vi "Wait for Operation Complete.vi"(2 "error in (no error)":errorcluster, 3 "Timeout (10000 ms)":u32=10000, 4 "VISA resource name":refnum<visa-resource-name>) -> (0 "error out":errorcluster, 1 "VISA resource name out":refnum<visa-resource-name>)   [LabVIEW 2020]
doc: "This low-level VI initiates a measurement. After you call this VI, the instrument leaves the idle state and waits for a trigger.\n\n<B>Note:</B> Use this VI only with other low-level VIs. The high-level VIs automatically incorporate this functionality. This VI does not check the instrument status. If you want to check the instrument status, call the Error Query VI at the conclusion of the sequence."
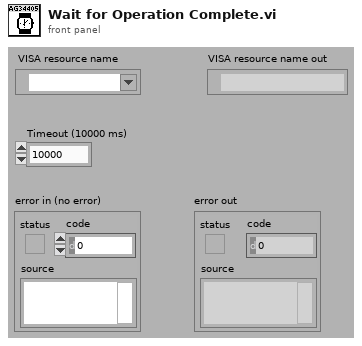
[diagram p1: front panel]
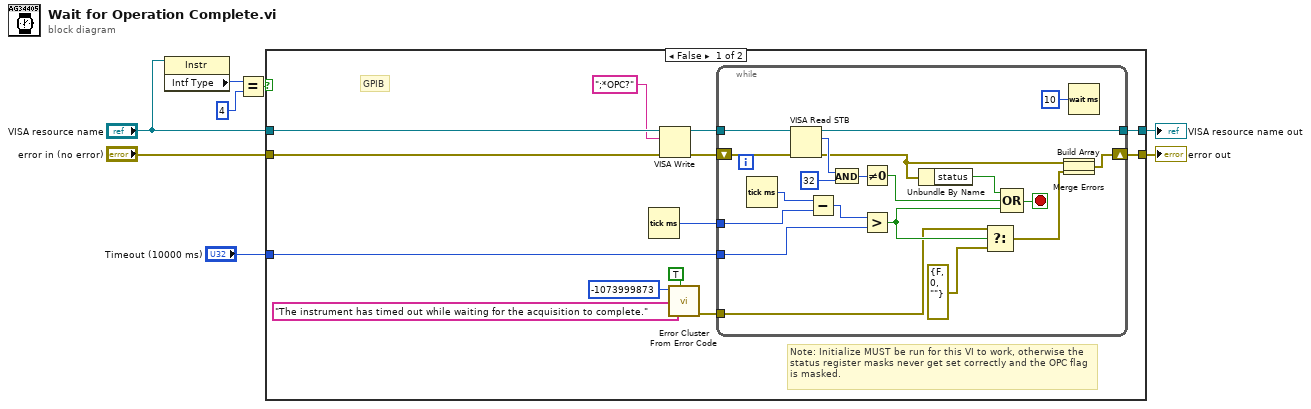
[diagram p0: block diagram]
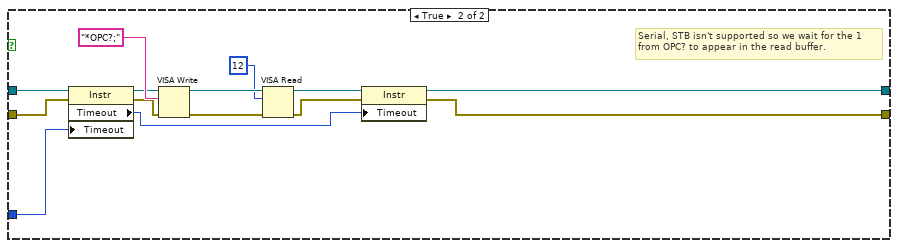
[diagram p2: hidden frame]
diagram:
  n1 = property class="Instr"(reference="VISA resource name") -> ("Intf Type"=w3:u16)  [unwired: 1 in, 2 out]
  n2 = Equal?(x=w3, y=u16 4) -> (x = y?=w4:bool)
  n3 = case shown="False" w4 {
    tunnel: "VISA resource name" -> [w21 w52]
    tunnel: "error in (no error)" -> [w20 w47]
    tunnel: [w17 w43] -> w7
    tunnel: [w16 w48] -> w6
    tunnel: "Timeout (10000 ms)" -> [w9 w51]
    frame False {
      # "GPIB"
      # "Note: Initialize MUST be run for this VI to work, otherwise the status register masks never get set correctly and the OPC flag is masked."
      n4 = Tick Count (ms)() -> (millisecond timer value=w14:u32)
      n5 = VISA Write(VISA resource name=w21, write buffer=";*OPC?", error in (no error)=w20) -> (VISA resource name out=w19:refnum<visa-resource-name>, error out=w18:errorcluster)  [unwired: 1 out]
      n6 = call <vilib>:"Error Cluster From Error Code.vi"("show call chain? (False)"=TRUE, "error message (\"\")"="The instrument has timed out while waiting for the acquisition to complete." ("error message (\"\")"), "error code (0)"=-1073999873) -> ("error out"=w10:errorcluster)  [unwired: 6 in]
      n7 = while {
        tunnel: w19 -> [w42]
        tunnel: [w40] -> w16
        tunnel: w14 -> [w35]
        shift-right: [w27] -> w17
        shift-left: w18 -> [w41]
        tunnel: w10 -> [w30]
        tunnel: w9 -> [w23]
        stop <- w32 stop-if-true
        n8 = Tick Count (ms)() -> (millisecond timer value=w36:u32)
        n9 = VISA Read STB(8:w41, 11:w42) -> (0:w26:errorcluster, 2:w39:u16, 3:w40:refnum<visa-resource-name>)
        n10 = Subtract(x=w36, y=w35) -> (x-y=w34:u32)
        n11 = And(x=w39, y=u16 32) -> (x .and. y?=w37:u16)
        n12 = Not Equal To 0?(x=w37) -> (x != 0?=w33:bool)
        n13 = Greater?(x=w34, y=w23) -> (0:w31:bool)
        n14 = Unbundle By Name(w26) -> ("status"=w25:bool)
        n15 = Select(t=w30, s=w31, f=errorcluster {"status"=FALSE, "code"=0, "source"=""}) -> (s? t:f=w28:errorcluster)
        n16 = Compound Arithmetic op=OR(w25, w33, w31) -> (w32:bool)
        n17 = Build Array(w26, w28) -> (w22:errorcluster[])
        n18 = Merge Errors(w22) -> (w27:errorcluster)
        n19 = Wait (ms)(milliseconds to wait=u32 10) -> ()  [unwired: 1 out]
      }
    }
    frame True {
      # "Serial, STB isn't supported so we wait for the 1 \nfrom OPC? to appear in the read buffer."
      n20 = property class="Instr"(reference=w52, error in=w47, "Timeout"=w51) -> (reference out=w46:refnum<visa-resource-name>, error out=w45:errorcluster, "Timeout"=w50:u32)
      n21 = VISA Write(VISA resource name=w46, write buffer="*OPC?;", error in (no error)=w45) -> (VISA resource name out=w54:refnum<visa-resource-name>, error out=w55:errorcluster)  [unwired: 1 out]
      n22 = VISA Read(VISA resource name=w54, byte count=u32 12, error in (no error)=w55) -> (VISA resource name out=w49:refnum<visa-resource-name>, error out=w44:errorcluster)  [unwired: 2 out]
      n23 = property class="Instr"(reference=w49, error in=w44, "Timeout"=w50) -> (reference out=w48:refnum<visa-resource-name>, error out=w43:errorcluster)
    }
  }
  "VISA resource name out" <- w6
  "error out" <- w7
